vi "PID Brake제어.vi"() -> ()   [LabVIEW 2016]
uses:
  <vilib>/Platform/TimedLoop/XDataNode/timing_clust.ctl
  <vilib>/Platform/TimedLoop/XDataNode/nitl_modes.ctl
  <vilib>/Platform/TimedLoop/XDataNode/wakeup.ctl
  <vilib>/addons/control/pid/pid.llb/PID (DBL).vi
  <vilib>/addons/control/pid/pid.llb/PID Lead-Lag (DBL).vi
  <vilib>/Platform/TimedLoop/XDataNode/XDataNode.xnode
  <vilib>/express/express arith-compare/Formula/XNode/ExpressFormulaBlockNode.xnode
  <vilib>/addons/control/pid/NI_PID_pid.lvlib
  <vilib>/Platform/TimedLoop/XDataNode/XDNodeRunTimeDep.lvlib
panel:
  in  "PID gains":T1={"proportional gain (Kc)"=1.0, "integral time (Ti, min)"=0.01, "derivative time (Td, min)"=0.0} caption="PID 게인" {"derivative time (Td, min)" format="%#.6g"; "integral time (Ti, min)" format="%#.6g"; "proportional gain (Kc)" format="%#.6g"}
  out "PV Setpoint Output":cluster{"initial PV":dbl, "setpoint":dbl}(graph)={"initial PV"=0.18693112703744846, "setpoint"=0.0}
  out "PID 입력 브레이크":dbl
  in  "PID 제동거리":dbl=0.5 format="%#_13g"
  out "Encoder Speed Filtered (m/s)":dbl
  out "입력된 속도(protocol)":dbl
  out "결과":dbl
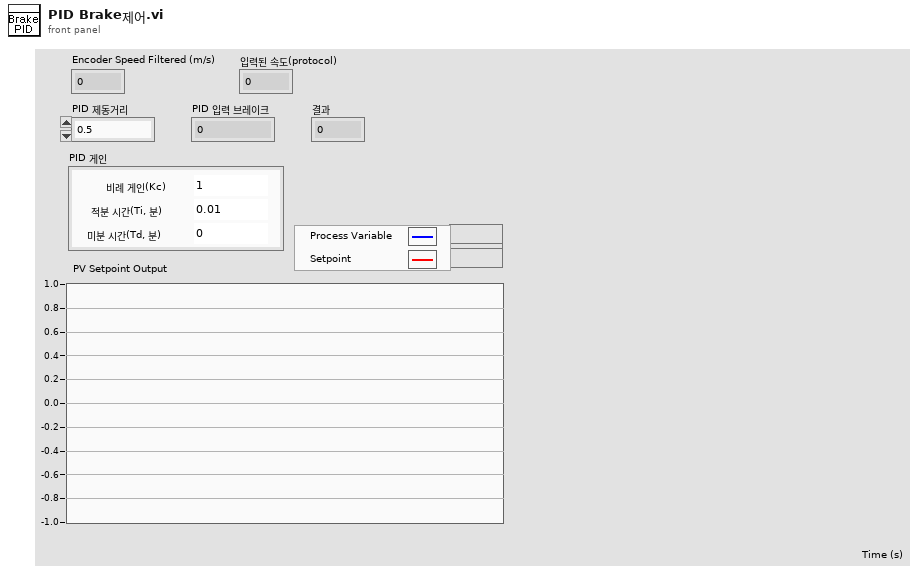
[diagram p1: front panel]
types:
  T1 = cluster{"proportional gain (Kc)":dbl, "integral time (Ti, min)":dbl, "derivative time (Td, min)":dbl}
  T2 = typedef "XDNodeRunTimeDep.lvlib/timing_clust.ctl" = cluster{"Expected End [f-1]":u64, "Actual End [f-1]":u64, "Finished Late? [f-1]":bool, "Expected End [i-1]":u64, "Actual End [i-1]":u64, "Finished Late? [i-1]":bool, "Expected Start [i]":u64, "Actual Start [i]":u64, "Expected Start [f]":u64, "Actual Start [f]":u64, "Source Name":string, "Structure Name":string, "Period":i64, "Deadline":i64, "Offset":i64, "Start":i64, "Priority":i32, "Timeout":i32, "Mode":T3, "Wakeup Reason":T4, "Error":errorcluster, "Source Type":string, "Secondary Source Type":string, "Global End Time":u64, "Global Start Time":u64, "Frame Duration":u64, "Iteration Duration":u64, "Assigned CPU":i32, "I/O Scan Engine Mode":u32}
  T3 = typedef "XDNodeRunTimeDep.lvlib/nitl_modes.ctl" = enum32{"No Change", "Process missed periods, maintain original phase", "Discard missed periods, maintain original phase", "Process missed periods, ignore original phase", "Discard missed periods, ignore original phase"}
  T4 = typedef "XDNodeRunTimeDep.lvlib/wakeup.ctl" = enum32{"Normal", "Aborted", "Asynchronous wakeup", "Timing source error", "Timed loop error", "Timeout"}
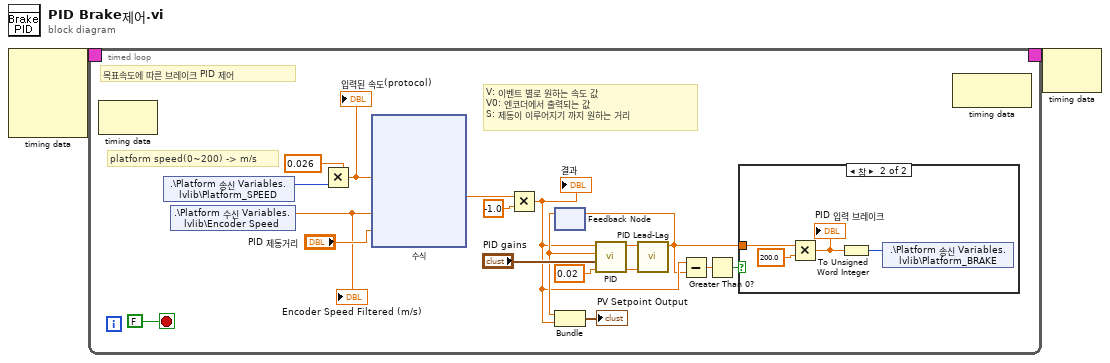
[diagram p0: block diagram]
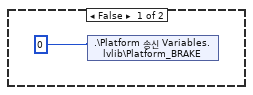
[diagram p2: hidden frame]
diagram:
  n1 = node-c288() -> (w2:T2)  [unwired: 4 in]
  n2 = timed-loop {
    timing: w2 -> [_]
    timing-out: [_] -> w1
    stop <- FALSE stop-if-true
    # "platform speed(0~200) -> m/s"
    # "목표속도에 따른 브레이크 PID 제어"
    # "V: 이벤트 별로 원하는 속도 값\nV0: 엔코더에서 출력되는 값\nS: 제동이 이루어지기 까지 원하는 거리"
    n3 = node-c288() -> ()  [unwired: 1 in, 1 out]
    n4 = shared-variable ".\\Platform 송신 Variables.lvlib\\Platform_SPEED"() -> (w4:u16)  [unwired: 1 in, 1 out]
    n5 = shared-variable ".\\Platform 수신 Variables.lvlib\\Encoder Speed"() -> (w3:dbl)  [unwired: 1 in, 1 out]
    "Encoder Speed Filtered (m/s)" <- w3
    n6 = Multiply(x=0.026, y=w4) -> (x*y=w7:dbl)
    "입력된 속도(protocol)" <- w7
    n7 = xnode "수식"("V"=w7, "V0"=w3, "S"="PID 제동거리") -> ("결과"=w12:dbl)  [unwired: 1 in, 1 out]
    n8 = Multiply(x=w12, y=-1.0) -> (x*y=w10:dbl)
    "결과" <- w10
    n9 = feedback #1() -> (w18:dbl)  [unwired: 1 in]
    n10 = Bundle("output"=w18, w10) -> (→"PV Setpoint Output":cluster{"output":dbl, dbl})  [unwired: 1 in]
    n11 = call-poly <vilib>:"PID.vi"("dt (s)"=0.02, "PID gains"="PID gains", "process variable"=w18, "setpoint"=w10) -> ("dt out (s)"=w16:dbl, "output"=w15:dbl)  [unwired: 6 in]
    n12 = call-poly <vilib>:"PID Lead-Lag.vi"("dt (s)"=w16, "input"=w15) -> ("output"=w9:dbl)  [unwired: 6 in, 1 out]
    n13 = feedback-in #1(w9) -> ()
    n14 = Subtract(x=w10, y=w9) -> (x-y=w8:dbl)
    n15 = Greater Than 0?(x=w8) -> (x > 0?=w11:bool)
    n16 = case shown="참" w11 {
      tunnel: w9 -> [_ w37]
      frame False {
        n17 = shared-variable ".\\Platform 송신 Variables.lvlib\\Platform_BRAKE"(i16 0 ("brake")) -> ()  [unwired: 1 in, 1 out]
      }
      frame True {
        n18 = Multiply(x=w37, y=200.0) -> (x*y=w35:dbl)
        "PID 입력 브레이크" <- w35
        n19 = To Unsigned Word Integer(number=w35) -> (unsigned 16bit integer=w34:u16)
        n20 = shared-variable ".\\Platform 송신 Variables.lvlib\\Platform_BRAKE"(w34) -> ()  [unwired: 1 in, 1 out]
      }
    }
    n21 = node-c288() -> ()  [unwired: 1 in, 1 out]
  }
  n22 = node-c288(w1) -> ()  [unwired: 1 out]
